vi "Wait for Shooter Ready.vi"(1 "Execute":bool=TRUE) -> (4 "Done Executing":bool)   [LabVIEW 2011]
uses:
  Globals/Shooter Speed Error.vi
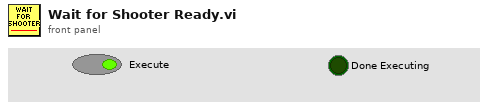
[diagram p1: front panel]
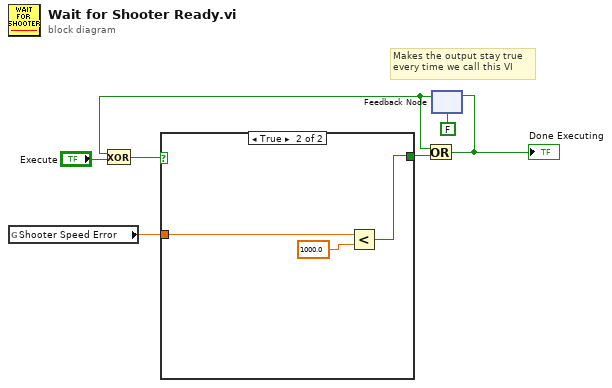
[diagram p0: block diagram]
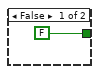
[diagram p2: hidden frame]
diagram:
  # "Makes the output stay true\nevery time we call this VI"
  n1 = global read "Shooter Speed Error.vi" "Shooter Speed Error"() -> (w1:dbl)
  n2 = feedback #1(FALSE) -> (w3:bool)
  n3 = Exclusive Or(1:"Execute", 2:w3) -> (0:w7:bool)
  n4 = case shown="True" w7 {
    tunnel: [FALSE w10] -> w5
    tunnel: w1 -> [_ w9]
    frame False {
    }
    frame True {
      n5 = Less?(x=w9, y=1000.0) -> (x < y?=w10:bool)
    }
  }
  n6 = Or(x=w3, y=w5) -> (x .or. y?=w2:bool)
  "Done Executing" <- w2
  n7 = feedback-in #1(w2) -> ()
